vi "KML-AddWPdata.vi"(10 "wp data in (raw)":string, 11 "kml file dir path":path) -> (2 "wpPlacemarkTxt":string)   [LabVIEW 8.6]
panel:
  # "Parse and Save WP Placemark Data"
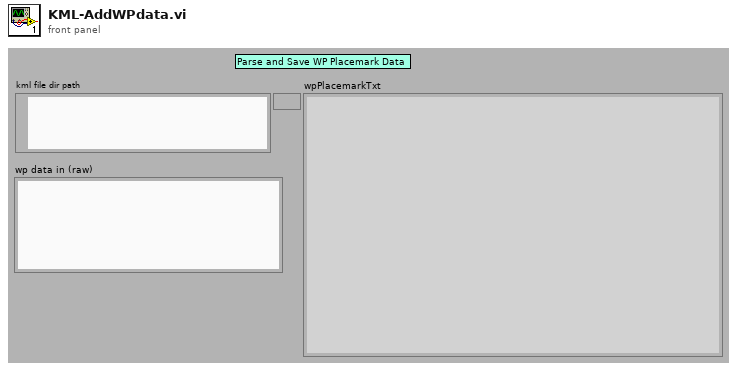
[diagram p1: front panel]
types:
  T1 = enum16{"open", "replace", "create", "open or create", "replace or create", "replace or create with confirmation"}
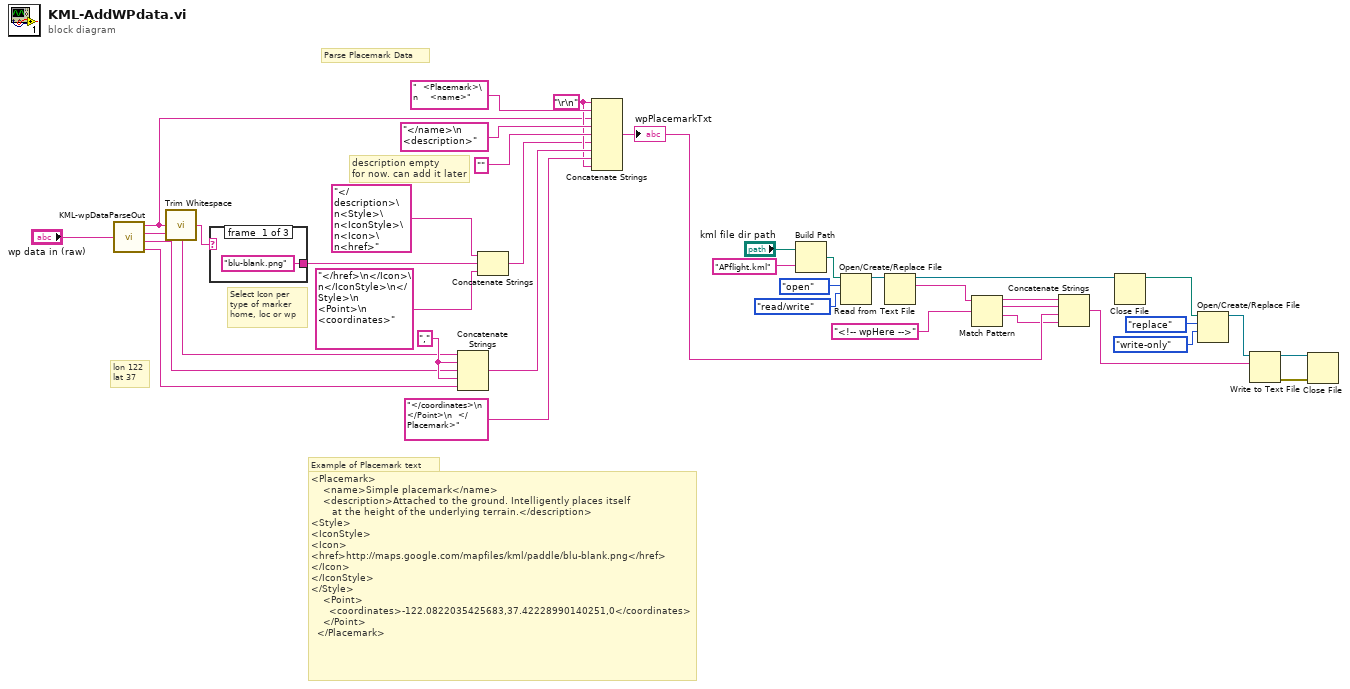
[diagram p0: block diagram]
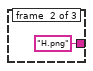
[diagram p2: hidden frame]
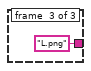
[diagram p3: hidden frame]
diagram:
  w31 = "\r\n"
  w34 = ","
  # "Select Icon per\ntype of marker\nhome, loc or wp"
  # "Parse Placemark Data"
  # "Example of Placemark text"
  # "lon 122\nlat 37"
  # "description empty\nfor now. can add it later"
  # "<Placemark>\n    <name>Simple placemark</name>\n    <description>Attached to the ground. Intelligently places itself \n       at the height of the underlying terrain.</description>\n<Style>\n<IconStyle>\n<Icon>\n<href>http://maps.google.com/mapfiles/kml/paddle/blu-blank.png</href>\n</Icon>\n</IconStyle>\n</Style>\n    <Point>\n      <coordinates>-122.0822035425683,37.42228990140251,0</coordinates>\n    </Point>\n  </Placemark>"
  n1 = call "KML-wpDataParseOut.vi"("wp data in"="wp data in (raw)") -> ("alt"=w27:string, "lat"=w28:string, "lon"=w29:string, "wp#"=w3:string)  [unwired: 4 in]
  n2 = call <vilib>:"Trim Whitespace.vi"("string"=w3) -> ("trimmed string"=w1:string)  [unwired: 1 in]
  n3 = case shown="\"loc\"" w1 {
    tunnel: ["blu-blank.png" "H.png" "L.png"] -> w2
    frame #0 {
    }
    frame #1 {
    }
    frame #2 {
    }
  }
  n4 = Concatenate Strings(w29, w34, w28, w34, w27) -> (w33:string)
  n5 = Concatenate Strings("</description>\n<Style>\n<IconStyle>\n<Icon>\n<href>", w2, "</href>\n</Icon>\n</IconStyle>\n</Style>\n    <Point>\n      <coordinates>") -> (w5:string)
  n6 = Concatenate Strings(w31, "  <Placemark>\n    <name>", w3, "</name>\n    <description>", "", w5, w33, "</coordinates>\n    </Point>\n  </Placemark>", w31) -> (w30:string)
  "wpPlacemarkTxt" <- w30
  n7 = Build Path(base path="kml file dir path", name or relative path="APflight.kml") -> (appended path=w22:path)
  n8 = Open/Create/Replace File(file path (use dialog)=w22, operation (0:open)=T1."open", access (0:read/write)=enum16{"read/write", "read-only", "write-only"}."read/write") -> (refnum out=w23:refnum<file>)  [unwired: 3 in, 2 out]
  n9 = Read from Text File(file (use dialog)=w23) -> (refnum out=w14:refnum<file>, text=w19:string)  [unwired: 3 in, 2 out]
  n10 = Match Pattern(string=w19, regular expression="<!-- wpHere -->") -> (before substring=w17:string, match substring=w16:string, after substring=w15:string)  [unwired: 1 in, 1 out]
  n11 = Concatenate Strings(w17, w16, w30, w15) -> (w10:string)
  n12 = Close File(refnum=w14) -> (path=w11:path)  [unwired: 1 in, 1 out]
  n13 = Open/Create/Replace File(file path (use dialog)=w11, operation (0:open)=T1."replace", access (0:read/write)=enum16{"read/write", "read-only", "write-only"}."write-only") -> (refnum out=w9:refnum<file>)  [unwired: 3 in, 2 out]
  n14 = Write to Text File(file (use dialog)=w9, text=w10) -> (refnum out=w8:refnum<file>, error out=w7:errorcluster)  [unwired: 2 in, 1 out]
  n15 = Close File(refnum=w8, error in=w7) -> ()  [unwired: 2 out]
